vi "Read Model.lvclass.vi"(8 "error in (no error)":errorcluster, 11 "PluginWithDatabase in":refnum<class "PluginWithDatabase.lvclass">) -> (0 "error out":errorcluster, 2 "UserManagement.lvlib:Model":refnum<class "Model.lvclass">, 3 "PluginWithDatabase out":refnum<class "PluginWithDatabase.lvclass">)   [LabVIEW 2015, in "ActorManagement.lvlib" / "PluginWithDatabase.lvclass"]
uses:
  PluginWithDatabase.lvclass
  UserManagement/Model/Model.lvclass
  PluginWithDatabase.lvclass/PluginWithDatabase.ctl
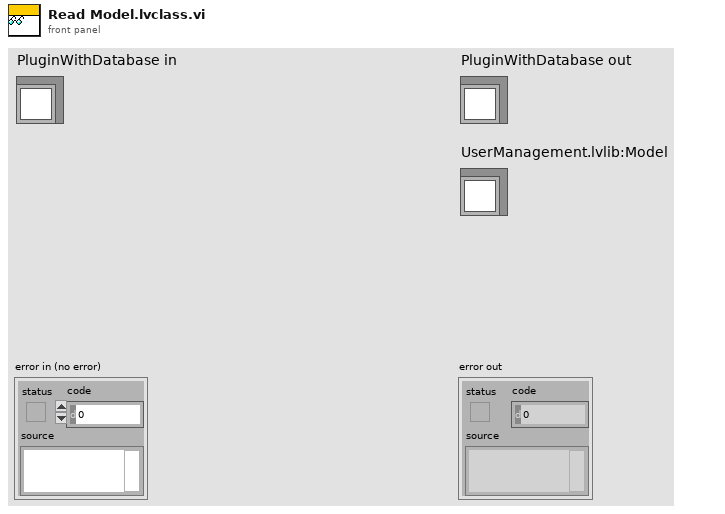
[diagram p1: front panel]
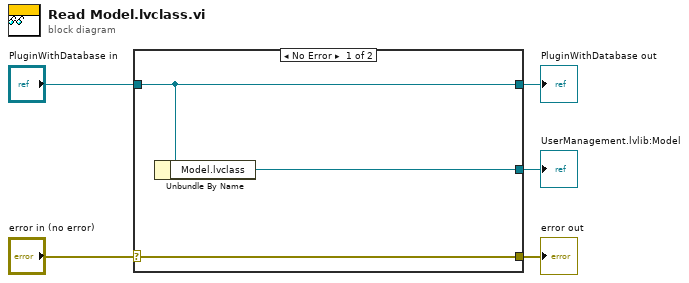
[diagram p0: block diagram]
diagram:
  n1 = case shown="No Error" "error in (no error)" {
    selector: "error in (no error)" -> [w8 w9]
    tunnel: [w8 w9] -> w4
    tunnel: [w7 w10] -> w2
    tunnel: "PluginWithDatabase in" -> [w7 w10]
    tunnel: [w6 _] -> w1
    frame No Error {
      n2 = Unbundle By Name(w7) -> ("Model.lvclass"=w6:refnum<class "Model.lvclass">)
    }
    frame Error {
    }
  }
  "error out" <- w4
  "PluginWithDatabase out" <- w2
  "UserManagement.lvlib:Model" <- w1
